vi "Set Compilation Notes.vi"(8 "error in (no error)":errorcluster, 9 "Notes":variant, 10 "note key":string, 11 "functionbase in":refnum<class "functionbase.lvclass">) -> (0 "error out":errorcluster, 3 "functionbase out":refnum<class "functionbase.lvclass">)   [LabVIEW 2019, in "LSL.lvlib" / "functionbase.lvclass"]
uses:
  functionbase.lvclass
  functionbase.lvclass/functionbase.ctl
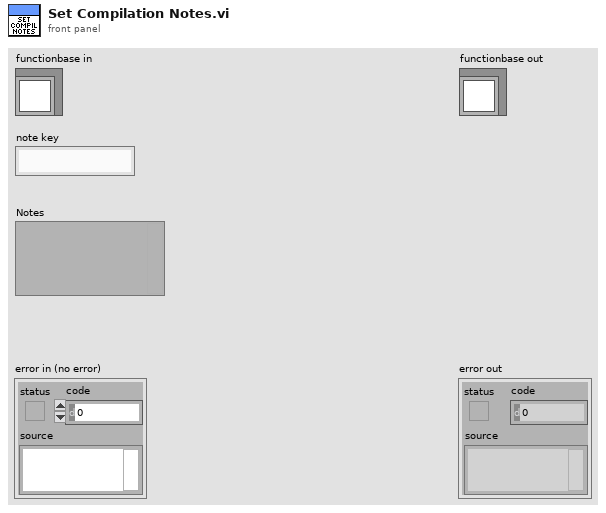
[diagram p1: front panel]
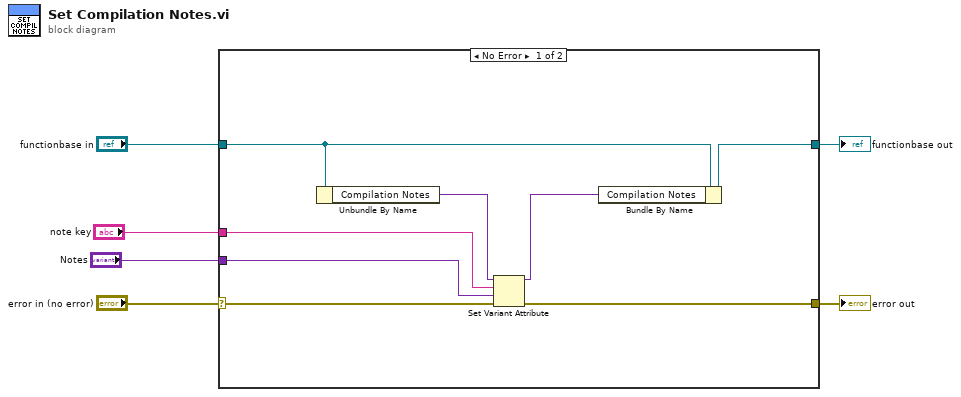
[diagram p0: block diagram]
diagram:
  n1 = case shown="No Error" "error in (no error)" {
    selector: "error in (no error)" -> [w13 w16]
    tunnel: [w12 w16] -> w5
    tunnel: [w7 w15] -> w3
    tunnel: "functionbase in" -> [w8 w15]
    tunnel: "note key" -> [w11 _]
    tunnel: "Notes" -> [w10 _]
    frame No Error {
      n2 = Unbundle By Name(w8) -> ("Compilation Notes"=w14:variant)
      n3 = Set Variant Attribute(Variant=w14, name=w11, value=w10, error in=w13) -> (Variant out=w9:variant, error out=w12:errorcluster)  [unwired: 1 out]
      n4 = Bundle By Name(cluster=w8, "Compilation Notes"=w9) -> (w7:refnum<class "functionbase.lvclass">)
    }
    frame Error {
    }
  }
  "error out" <- w5
  "functionbase out" <- w3
